vi "Allocate Intermediate Buffer.vi"(8 "error in (no error)":errorcluster, 10 "unallocated Intermediate Buffer":refnum<class "Double Pointer.lvclass">, 11 "Framework in":refnum<class "VeriStand DSF.Framework.lvclass">) -> (0 "error out":errorcluster, 2 "allocated Intermediate Buffer":refnum<class "Double Pointer.lvclass">, 3 "Framework out":refnum<class "VeriStand DSF.Framework.lvclass">)   [LabVIEW 2017, in "Data Sharing Framework Engine.lvlib" / "VeriStand DSF.Framework.lvclass"]
uses:
  VeriStand DSF.Framework.lvclass
  Builds/Current/Data Sharing Framework Core/Data Sharing Framework Core.lvlibp/Engine/Internal/Memory/Double Pointer/Double Pointer.lvclass
  C:/github/data-sharing-framework/Data Sharing Framework/Builds/Current/Data Sharing Framework Core/Data Sharing Framework Core.lvlibp/1abvi3w/vi.lib/National Instruments/Memory Manager/Classes/Pointer/Memory.Pointer.lvclass
  Builds/Current/Data Sharing Framework Core/Data Sharing Framework Core.lvlibp/Engine/Framework/Framework.lvclass
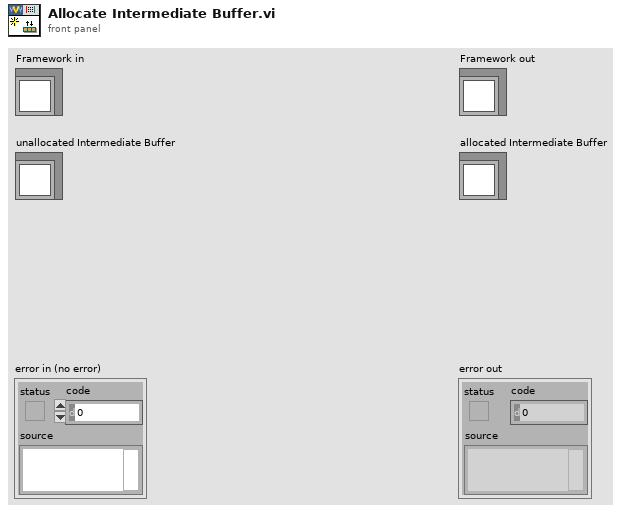
[diagram p1: front panel]
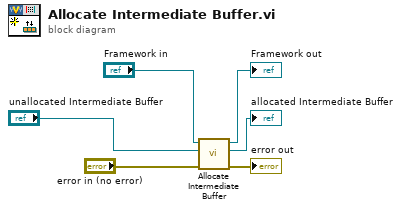
[diagram p0: block diagram]
diagram:
  n1 = call-parent "Allocate Intermediate Buffer.vi"("error in (no error)"="error in (no error)", "unallocated Intermediate Buffer"="unallocated Intermediate Buffer", "Framework in"="Framework in") -> ("error out"=→"error out":errorcluster, "allocated Intermediate Buffer"=→"allocated Intermediate Buffer":refnum<class "DSF.Engine.Pointer.DBL.lvclass">, "Framework out"=→"Framework out":refnum<class "VeriStand DSF.Framework.lvclass">)  [unwired: 6 in]
